vi "NewBlockOnTheBlock.vi"(8 "Numeric 2":dbl, 11 "Numeric":dbl) -> (3 "Motor Values":dbl[](array[numeric]))   [LabVIEW 2015]
uses:
  <vilib>/Rock Robotics/WPI/Utilities/WPI_GetSetVariantRefNum.vi
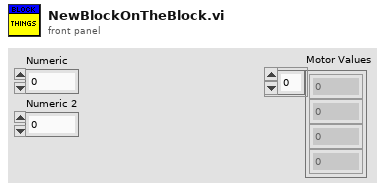
[diagram p1: front panel]
types:
  T1 = typedef "WPI_RobotDriveDevRef.ctl" = cluster{"DevStatus":errorcluster, "Motors[]":T2[], "Square Inputs":bool, "Max Output":dbl}
  T2 = typedef "WPI_MotorControlDeviceRef.ctl" = cluster{"DeviceStatus":errorcluster, "Type":T3, "PWM":cluster{"PWM Channel":T4, "DeadBand":T5}, "CAN":cluster{"Device Number":u8, "Control Mode":T6, "Semaphore":T7, "Max Vout":dbl, "TalonSRX Control Mode":T8}, "Invert":bool}
  T3 = typedef "WPI_MotorControlType.ctl" = enum16{"PWM", "CAN", "CANTalonSRX"}
  T4 = typedef "FPGA_DIOPWMChannel.ctl" = enum8{"PWM 0", "PWM 1", "PWM 2", "PWM 3", "PWM 4", "PWM 5", "PWM 6", "PWM 7", "PWM 8", "PWM 9", "PWM MXP 0", "PWM MXP 1", "PWM MXP 2", "PWM MXP 3", "PWM MXP 4", "PWM MXP 5", "PWM MXP 6", "PWM MXP 7", "PWM MXP 8", "PWM MXP 9", "Invalid"}
  T5 = typedef "WPI_PWMDeadband.ctl" = cluster{"Name":string, "maxPositivePwm":i32, "minPositivePwm":i32, "centerPwm":i32, "maxNegativePwm":i32, "minNegativePwm":i32, "angularRange":u16}
  T6 = typedef "WPI_CANJaguar_ControlMode.ctl" = enum8{"Percent VBus", "Current", "Speed", "Position", "Voltage"}
  T7 = typedef "Semaphore RefNum" = refnum<k1>
  T8 = typedef "WPI_CANTalonSRX_APIControlMode.ctl" = enum8{"Percent VBus", "Speed", "Position", "Slave", "Unchanged / Invalid", "Voltage Compensation", "Current", "Motion Profile"}
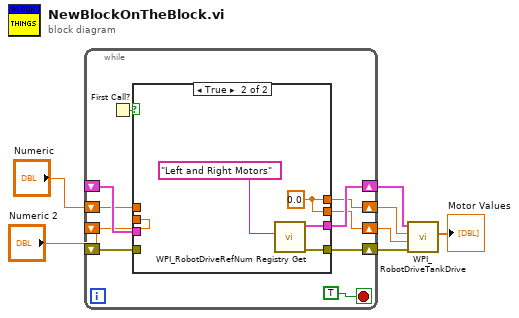
[diagram p0: block diagram]
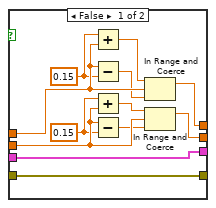
[diagram p2: hidden frame]
diagram:
  n1 = while {
    shift-right: [w15] -> w7
    shift-left: _ -> [w11]
    shift-right: [w14] -> w6
    shift-left: _ -> [w10]
    shift-right: [w13] -> w5
    shift-left: "Numeric" -> [w9]
    shift-right: [w12] -> w4
    shift-left: "Numeric 2" -> [w8]
    stop <- TRUE stop-if-true
    n2 = First Call?() -> (First Call?: T/F=w16:bool)
    n3 = case shown="True" w16 {
      tunnel: [w29 w32] -> w15
      tunnel: [w18 w31] -> w14
      tunnel: [w19 w30] -> w13
      tunnel: [w20 w30] -> w12
      tunnel: w11 -> [w29 _]
      tunnel: w10 -> [w18 _]
      tunnel: w9 -> [w27 _]
      tunnel: w8 -> [w23 _]
      frame False {
        w25 = 0.15 ("x")
        w22 = 0.15 ("x")
        n4 = Add(x=w25, y=w27) -> (x+y=w28:dbl)
        n5 = Subtract(x=w27, y=w25) -> (x-y=w26:dbl)
        n6 = Add(x=w22, y=w23) -> (x+y=w24:dbl)
        n7 = Subtract(x=w23, y=w22) -> (x-y=w21:dbl)
        n8 = In Range and Coerce(upper limit=w28, x=w27, lower limit=w26) -> (coerced(x)=w19:dbl)  [unwired: 1 out]
        n9 = In Range and Coerce(upper limit=w24, x=w23, lower limit=w21) -> (coerced(x)=w20:dbl)  [unwired: 1 out]
      }
      frame True {
        w30 = 0.0
        n10 = call <vilib>:"WPI_RobotDriveRefNum Registry Get.vi"("refnum name"="Left and Right Motors") -> ("error out"=w31:errorcluster, "RobotDriveDevRef"=w32:T1)  [unwired: 9 in]
      }
    }
  }
  n11 = call <vilib>:"WPI_RobotDriveTankDrive.vi"("error in (no error)"=w6, "Right axis value"=w4, "Left axis value"=w5, "RobotDriveDevRef"=w7) -> ("Motor Values"=→"Motor Values":dbl[])  [unwired: 5 in, 2 out]
